vi "Finding First Operator.vi"(8 "error in":errorcluster, 10 "String In":string) -> (0 "error out":errorcluster, 1 "Right String Out":string, 2 "First Operator Out":refnum<class "Formula Phrasing Binary Tree Node.lvclass">, 3 "Left String Out":string)   [LabVIEW 2024, in "Formula String Spliter Library.lvlib"]
uses:
  Formula String Spliter Library.lvlib
  Formula Phrasing Binary Tree Node/Formula Phrasing Binary Tree Node.lvclass
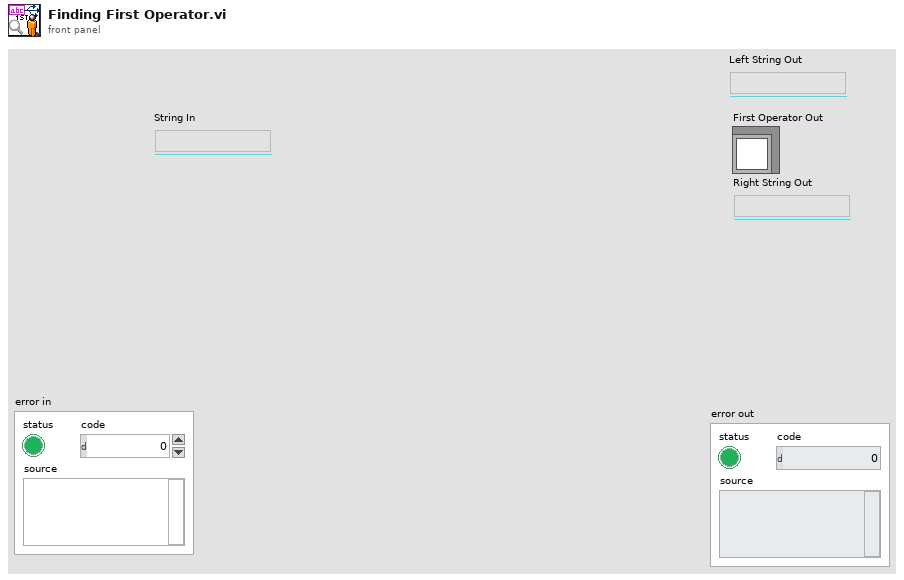
[diagram p1: front panel]
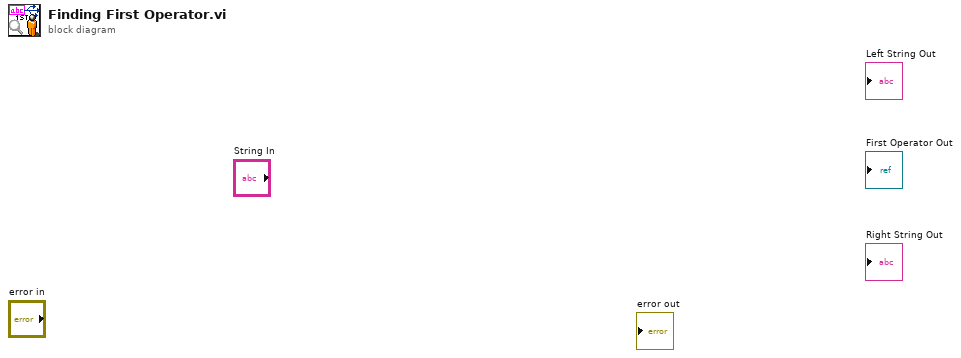
[diagram p0: block diagram]
diagram:
